vi "Check the Symbols.vi"(0 "Item Symbols":i32[](array[numeric])) -> (4 "All Selected?":bool, 6 "None Selected":bool)   [LabVIEW 2021, in "Packager Helpers.lvlib"]
uses:
  Packager Helpers.lvlib
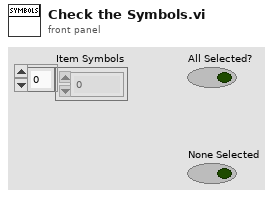
[diagram p1: front panel]
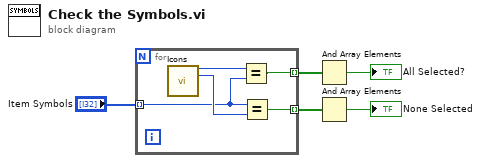
[diagram p0: block diagram]
diagram:
  n1 = for {
    tunnel: [w10] -> w4 mode=indexing
    tunnel: [w9] -> w5 mode=indexing
    tunnel: "Item Symbols" -> [w6] mode=indexing
    n2 = call "Icons.vi"() -> ("Selected"=w8:i32, "Non Selected"=w7:i32)  [unwired: 14 in]
    n3 = Equal?(x=w8, y=w6) -> (x = y?=w10:bool)
    n4 = Equal?(x=w6, y=w7) -> (x = y?=w9:bool)
  }
  n5 = And Array Elements(Boolean array=w4) -> (logical AND=→"All Selected?":bool)
  n6 = And Array Elements(Boolean array=w5) -> (logical AND=→"None Selected":bool)
